vi "motorsGlobalVar.vi"() -> ()   [LabVIEW 2014]
panel:
  in  "STOP application":bool
  in  "Motor Global Var":dbl[][](array[numeric]) format="%#_10g"
  # "These are absolute positions"
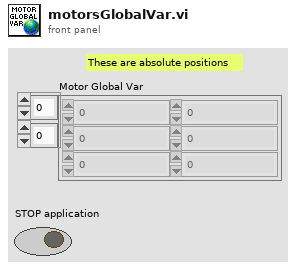
[diagram p1: front panel]
diagram:
